vi "RotationMatrix6DOF.vi"(1 "Eta":dbl[](array[numeric])) -> (0 "R":dbl[][](array[numeric]))   [LabVIEW 2014]
uses:
  <vilib>/imath/engines/lvmath2/RunTimeEngine/IndexRead/NIMS V(S).vi
  <instcachedir>/0/NIMS V(S)_0488751826AF41519A22953C041130DC.lvgen/NIMS V(S)_0488751826AF41519A22953C041130DC_000.vi
  <vilib>/imathl/engines/lvmath/Functions/Error Handling/Create Error.vi
  <vilib>/imath/engines/lvmath2/RunTimeEngine/NodeEndStatement/NIMS_NodeEndStatement_Output.vi
  <instcachedir>/0/NIMS_NodeEndStatement_Output_53EC0D466D134D7ABD903AC30B43404B.lvgen/NIMS_NodeEndStatement_Output_53EC0D466D134D7ABD903AC30B43404B_002.vi
  <vilib>/imath/engines/lvmath2/RunTimeEngine/ErrorHandling/NIMS_Finalize Error.vi
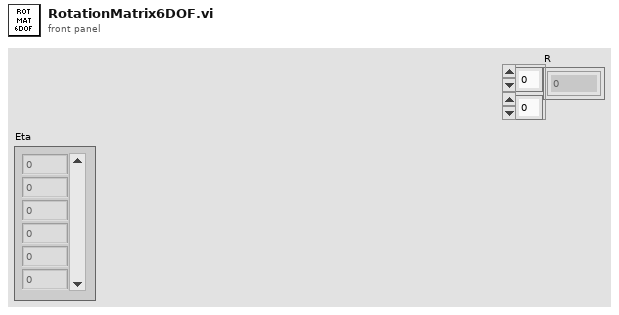
[diagram p1: front panel]
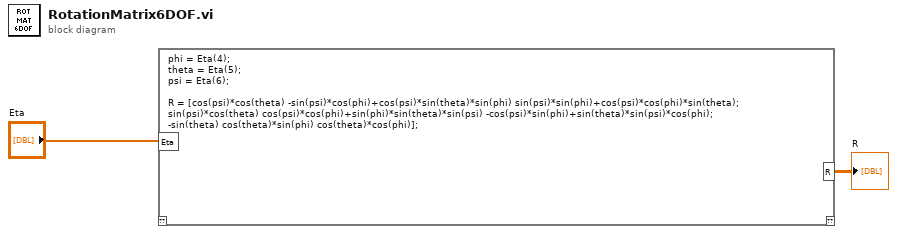
[diagram p0: block diagram]
diagram:
  n1 = mathscript code="phi = Eta(4);\ntheta = Eta(5);\npsi = Eta(6);\n\nR = [cos(psi)*cos(theta) -sin(psi)*cos(phi)+cos(psi)*sin(theta)*sin(phi) sin(psi)*sin(phi)+cos(psi)*cos(phi)*sin(theta);\nsin(psi)*cos(theta) cos(psi)*cos(phi)+sin(phi)*sin(theta)*sin(psi) -cos(psi)*sin(phi)+sin(theta)*sin(psi)*cos(phi);\n-sin(theta) cos(theta)*sin(phi) cos(theta)*cos(phi)];"("Eta"="Eta") -> ("R"=→"R":dbl[][])  [unwired: 1 in, 1 out]
